vi "ExperimentNo.vi"(8 "error in (no error)":errorcluster, 9 "Python version":string="3.7", 11 "user.xls path":path) -> (0 "error out":errorcluster, 2 "total":i32, 3 "experiment_No":i32)   [LabVIEW 2020]
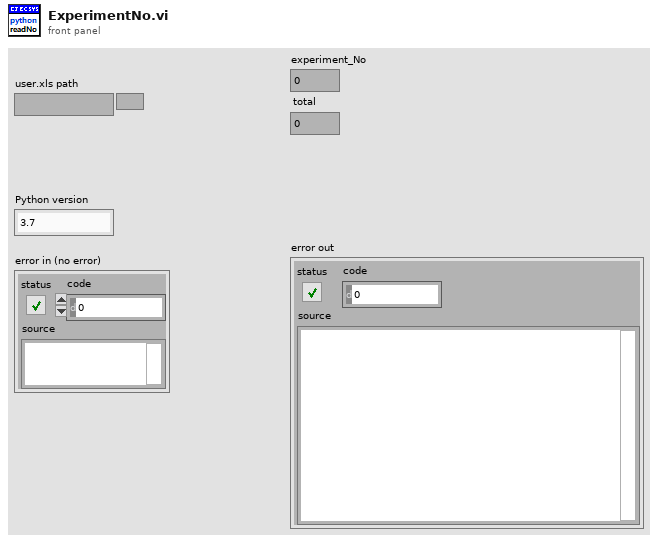
[diagram p1: front panel]
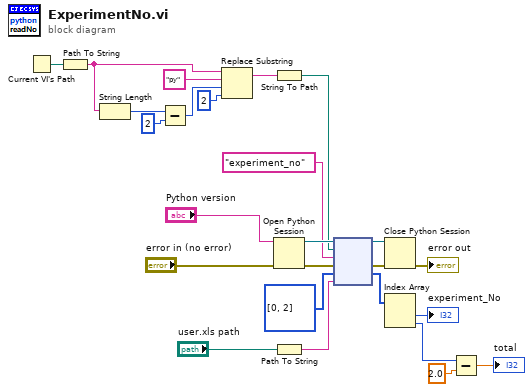
[diagram p0: block diagram]
diagram:
  n1 = Current VI's Path() -> (path=w15:path)
  n2 = Path To String(path=w15) -> (string=w14:string)
  n3 = String Length(string=w14) -> (length=w11:i32)
  n4 = Subtract(x=w11, y=2) -> (x-y=w10:i32)
  n5 = Replace Substring(2:2 ("length (len. of substring)"), 3:w10, 4:"py" ("substring (\"\")"), 5:w14) -> (1:w8:string)  [unwired: 1 out]
  n6 = String To Path(string=w8) -> (path=w7:path)
  n7 = Open Python Session(python version="Python version", 3:"error in (no error)") -> (session out=w24:refnum<k35>, error out=w21:errorcluster)  [unwired: 1 in]
  n8 = Path To String(path="user.xls path") -> (string=w17:string)
  n9 = node(w24, w7, "experiment_no" ("function name"), w21, i32[] [0, 2], w17) -> (w23:refnum<k35>, w22:errorcluster, w5:i32[])  [unwired: 1 in, 2 out]
  n10 = Close Python Session(session in=w23, error in=w22) -> (11:→"error out":errorcluster)
  n11 = Index Array(array=w5) -> (element #1=→"experiment_No":i32, element #2=w2:i32)  [unwired: 2 in]
  n12 = Subtract(x=w2, y=2.0) -> (x-y=→"total":dbl)
